vi "VsEPCal-Get Metrics.vi"(8 "error in (no error)":errorcluster, 10 "#AVERAGES":i32=1, 11 "Data in":dbl[](array[numeric])) -> (0 "error out":errorcluster, 2 "accelerometer (mV)":dbl, 3 "Data out":dbl[](array[numeric]))   [LabVIEW 2020]
uses:
  <vilib>/Analysis/baseanly.llb/Mean (DBL).vi
  <vilib>/Analysis/NI_AALBase.lvlib
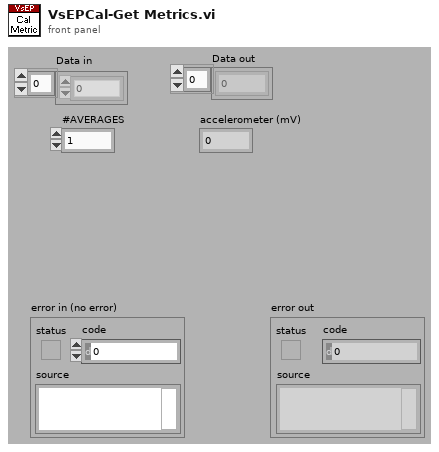
[diagram p1: front panel]
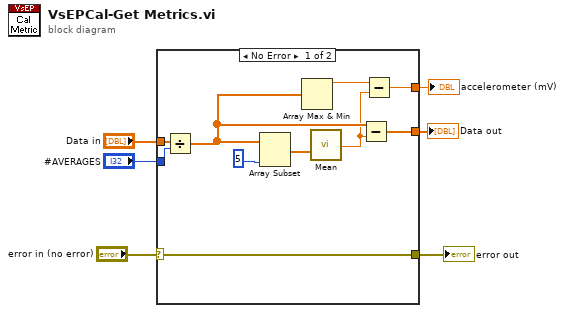
[diagram p0: block diagram]
diagram:
  n1 = case shown="No Error" "error in (no error)" {
    selector: "error in (no error)" -> [w11 w17]
    tunnel: "Data in" -> [w14 _]
    tunnel: "#AVERAGES" -> [w13 _]
    tunnel: [w12 _] -> w4
    tunnel: [w11 w17] -> w2
    tunnel: [w7 _] -> w1
    frame No Error {
      n2 = Divide(x=w14, y=w13) -> (x/y=w10:dbl[])
      n3 = Array Subset(array=w10, length=5) -> (w15:dbl[])  [unwired: 1 in]
      n4 = Array Max & Min(array=w10) -> (max value=w9:dbl)  [unwired: 3 out]
      n5 = call-poly <vilib>:"Mean.vi"("X"=w15) -> ("mean"=w8:dbl)  [unwired: 1 out]
      n6 = Subtract(x=w10, y=w8) -> (x-y=w12:dbl[])
      n7 = Subtract(x=w9, y=w8) -> (x-y=w7:dbl)
    }
    frame Error {
    }
  }
  "Data out" <- w4
  "accelerometer (mV)" <- w1
  "error out" <- w2
